vi "Z Aux Direct Connreframe.vi"(6 "piAxislist":i32, 7 "imaxaxises":i32, 8 "error in (no error)":errorcluster caption="错误输入（无错误）", 9 "tablenum":i32, 10 "frame":i32, 11 "handle":u32) -> (0 "error out":errorcluster caption="错误输出", 2 "function return":i32, 3 "handle out":u32, 4 "piAxislist out":i32)   [LabVIEW 2015, in "zauxdll.lvlib"]
doc: "int32 __stdcall ZAux_Direct_Connreframe(ZMC_HANDLE handle, int frame, int tablenum , int imaxaxises , int *piAxislist);"
uses:
  zauxdll.lvlib
  zauxdll.dll
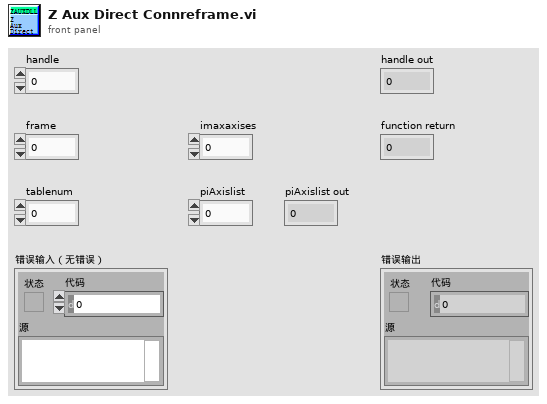
[diagram p1: front panel]
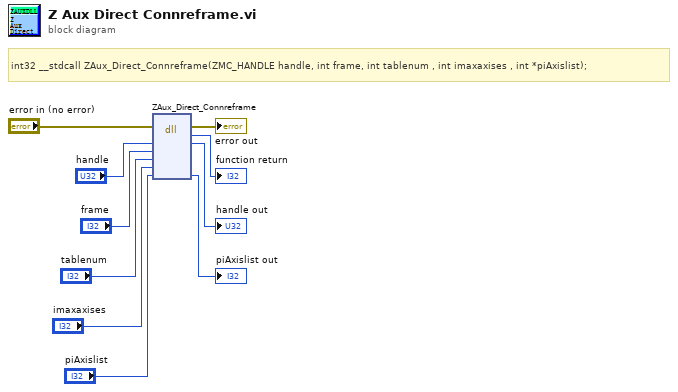
[diagram p0: block diagram]
diagram:
  # "int32 __stdcall ZAux_Direct_Connreframe(ZMC_HANDLE handle, int frame, int tablenum , int imaxaxises , int *piAxislist);"
  n1 = dll-call lib="C:/Users/VIC/Desktop/GOGORO_Oringnal - Panasonic/system/LLB/zmotion/zaux/zauxdll.*" fn="ZAux_Direct_Connreframe"(error in="error in (no error)", "handle"="handle", "frame"="frame", "tablenum"="tablenum", "imaxaxises"="imaxaxises", "piAxislist"="piAxislist") -> (error out=→"error out":errorcluster, →"function return":i32, "handle"=→"handle out":u32, "piAxislist"=→"piAxislist out":i32)  [unwired: 5 in, 1 out]
